vi "WriteBase.vi"(0 "Konvolucio MCAN120803 Adapter Class in":refnum<class "Konvolucio MCAN120803 Adapter Class.lvclass">, 5 "Id":u32 format="%08x", 7 "DataLength":i32, 9 "Data":u8[](array[numeric]) format="%02x", 11 "error in (no error)":errorcluster) -> (4 "Konvolucio MCAN120803 Adapter Class out":refnum<class "Konvolucio MCAN120803 Adapter Class.lvclass">, 15 "error out":errorcluster)   [LabVIEW 2011, in "Konvolucio MCAN120803 Adapter Class.lvclass"]
uses:
  Konvolucio MCAN120803 Adapter Class.lvclass
  Konvolucio MCAN120803 Adapter Class.lvclass/Konvolucio MCAN120803 Adapter Class.ctl
  <instrlib>/Konvolucio MCAN120803/Konvolucio MCAN120803.lvlib
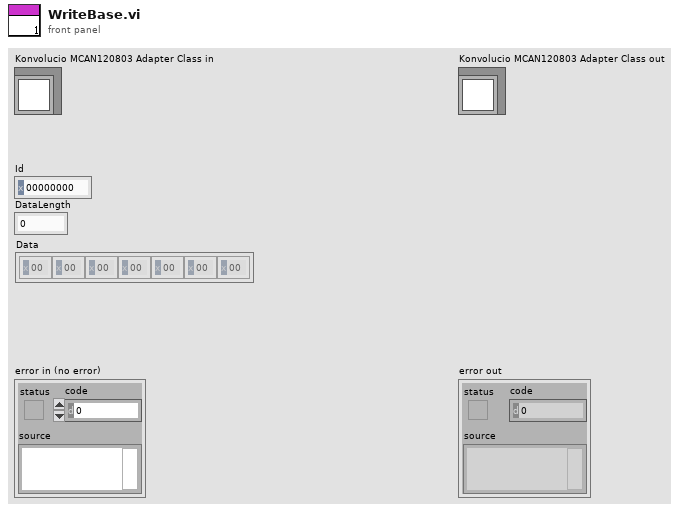
[diagram p1: front panel]
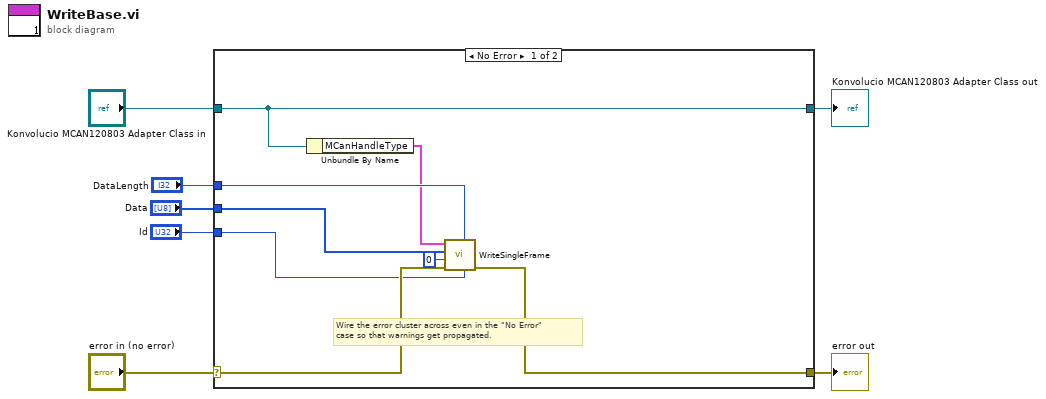
[diagram p0: block diagram]
diagram:
  n1 = case shown="No Error" "error in (no error)" {
    selector: "error in (no error)" -> [w15 w17]
    tunnel: [w14 w17] -> w6
    tunnel: [w10 w16] -> w4
    tunnel: "Konvolucio MCAN120803 Adapter Class in" -> [w10 w16]
    tunnel: "Data" -> [w13 _]
    tunnel: "DataLength" -> [w12 _]
    tunnel: "Id" -> [w11 _]
    frame No Error {
      # "Wire the error cluster across even in the \"No Error\"\ncase so that warnings get propagated."
      n2 = Unbundle By Name(w10) -> ("MCanHandleType"=w9:cluster{"MCanAdapter":refnum<k24>})
      n3 = call <instrlib>:"WriteSingleFrame.vi"("ArbitrationId"=w11, "DataLength"=w12, "error in"=w15, "IsRemote"=u8 0, "Data"=w13, "CanHandleIn"=w9) -> ("error out"=w14:errorcluster)  [unwired: 4 in, 1 out]
    }
    frame Error {
    }
  }
  "error out" <- w6
  "Konvolucio MCAN120803 Adapter Class out" <- w4
